vi "Read Data.vi"(0 "comm interface in":refnum<class "RoboRIO SPI.lvclass">, 5 "bytes to read":i32, 11 "error in":errorcluster) -> (4 "comm interface out":refnum<class "RoboRIO SPI.lvclass">, 6 "data":u8[](array[numeric]), 15 "error out":errorcluster)   [LabVIEW 2018, in "RoboRIO SPI.lvclass"]
uses:
  RoboRIO SPI.lvclass
  RoboRIO SPI.lvclass/RoboRIO SPI.ctl
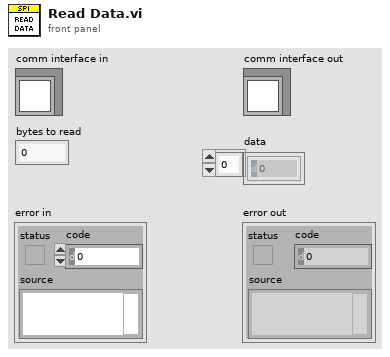
[diagram p1: front panel]
types:
  T1 = typedef "WPI_SPIDevRef.ctl" = cluster{"DevStatus":errorcluster, "Handle":i32, "SPI Bus":T2}
  T2 = typedef "spi_bus.ctl" = enum16{"SPI On-Board, CS0", "SPI On-Board, CS1", "SPI On-Board, CS2", "SPI On-Board, CS3", "SPI MXP", "Invalid"}
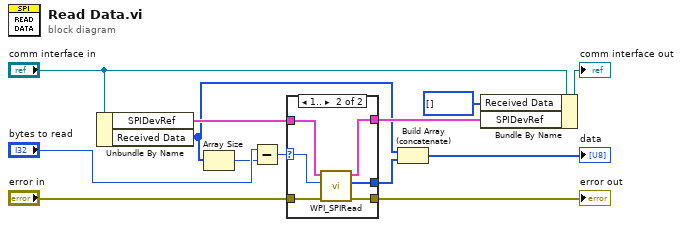
[diagram p0: block diagram]
diagram:
  n1 = Unbundle By Name("comm interface in") -> ("SPIDevRef"=w12:T1, "Received Data"=w4:u8[])
  n2 = Array Size(array=w4) -> (size(s)=w6:i32)
  n3 = Subtract(x="bytes to read", y=w6) -> (x-y=w5:i32)
  n4 = case shown="1.." w5 {
    selector: w5 -> [_ w17]
    tunnel: "error in" -> [w14 w21]
    tunnel: w12 -> [w15 w20]
    tunnel: [w15 w19] -> w9
    tunnel: [w14 w18] -> w8
    tunnel: [_ w16] -> w3
    frame ..0 {
    }
    frame 1.. {
      n5 = call <vilib>:"WPI_SPIRead.vi"("error in (no error)"=w21, "Num to Read"=w17, "SPIDevRef"=w20) -> ("error out"=w18:errorcluster, "Received Data"=w16:u8[], "SPIDevRef"=w19:T1)  [unwired: 6 in]
    }
  }
  "error out" <- w8
  n6 = Build Array (concatenate)(w4, w3) -> (→"data":u8[])
  n7 = Bundle By Name(cluster="comm interface in", "Received Data"=u8[] [], "SPIDevRef"=w9) -> (→"comm interface out":refnum<class "RoboRIO SPI.lvclass">)
